vi "Q Top Level.vi"() -> ()   [LabVIEW 2021, in "Qs.lvlib"]
uses:
  Qs.lvlib
panel:
  in  "Numeric Control":i32
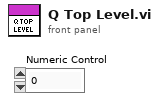
[diagram p1: front panel]
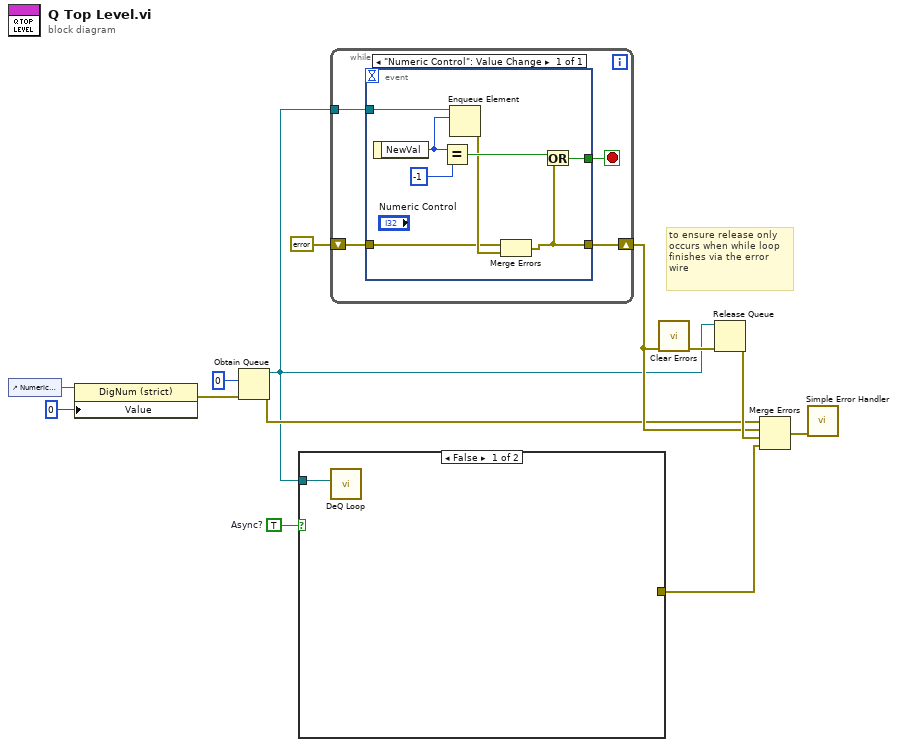
[diagram p0: block diagram]
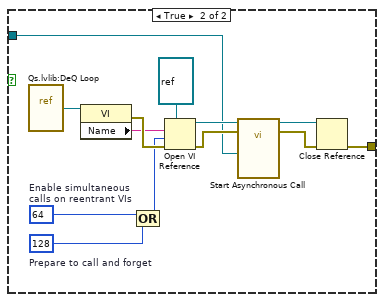
[diagram p2: hidden frame]
diagram:
  w3 = TRUE  # Async?
  # "to ensure release only occurs when while loop finishes via the error wire"
  n1 = control-ref of="Numeric Control"() -> (w13:refnum<vi>)
  n2 = property class="DigNum (strict)"(reference=w13, "Value"=0) -> (error out=w9:errorcluster)  [unwired: 1 in, 1 out]
  n3 = Obtain Queue(element data type=0 ("I32"), error in (no error)=w9) -> (queue out=w2:refnum<queue>, error out=w4:errorcluster)  [unwired: 3 in, 1 out]
  n4 = case shown="False" w3 {
    tunnel: w2 -> [w14 w16]
    tunnel: [_ w15] -> w1
    frame False {
      n5 = call "DeQ Loop.vi"("Queue"=w14) -> ()  [unwired: 11 in]
    }
    frame True {
      w22 = 128  # Prepare to call and forget
      w23 = 64  # Enable simultaneous calls on reentrant VIs
      n6 = vi-ref "Qs.lvlib:DeQ Loop.vi"() -> (w26:refnum<vi>)
      n7 = property class="VI"(reference=w26) -> (error out=w25:errorcluster, "Name"=w24:string)  [unwired: 1 in, 1 out]
      n8 = Compound Arithmetic op=OR(w23, w22) -> (w21:i32)
      n9 = Open VI Reference(type specifier VI Refnum (for type only)=refnum<vi> refnum, vi path=w24, options=w21, error in (no error)=w25) -> (vi reference=w19:refnum<vi>, error out=w20:errorcluster)  [unwired: 2 in]
      n10 = call-by-ref "Start Asynchronous Call"(reference=w19, error in=w20, "Queue"=w16) -> (reference out=w17:refnum<vi>, error out=w18:errorcluster)  [unwired: 11 in]
      n11 = Close Reference(reference=w17, error in (no error)=w18) -> (error out=w15:errorcluster)
    }
  }
  n12 = while {
    shift-right: [w30] -> w5
    shift-left: errorcluster {"status"=FALSE, "code"=0, "source"=""} ("error IO") -> [w29]
    tunnel: w2 -> [w28]
    stop <- w31 stop-if-true
    n13 = event shown="[0] \"Numeric Control\": Value Change" {
      selector: _ -> [_]
      dyn-events: _ -> [_]
      timeout: _ -> [_]
      tunnel: w28 -> [w36]
      tunnel: [w33] -> w31
      tunnel: [w32] -> w30
      tunnel: w29 -> [w34]
      event "Numeric Control": Value Change {
        n14 = event-data() -> ("NewVal"=w37:i32)  [unwired: 1 in]
        n15 = Equal?(x=w37, y=-1) -> (x = y?=w38:bool)
        n16 = Enqueue Element(queue=w36, element=w37) -> (error out=w35:errorcluster)  [unwired: 2 in, 2 out]
        n17 = Merge Errors(w34, w35) -> (w32:errorcluster)
        n18 = Or(x=w38, y=w32) -> (x .or. y?=w33:bool)
      }
    }
  }
  n19 = call <vilib>:"Clear Errors.vi"("error in (no error)"=w5) -> ("error out"=w6:errorcluster)  [unwired: 5 in, 1 out]
  n20 = Release Queue(queue=w2, error in (no error)=w6) -> (error out=w7:errorcluster)  [unwired: 1 in, 2 out]
  n21 = Merge Errors(w4, w5, w7, w1) -> (w10:errorcluster)
  n22 = call <vilib>:"Simple Error Handler.vi"("error in (no error)"=w10) -> ()  [unwired: 4 in, 5 out]
